vi "bad apple.vi"() -> ()   [LabVIEW 2016]
uses:
  <vilib>/vision/NI_Vision_Development_Module.lvlib
panel:
  out "强度图":sgl[][](graph)
  out "Image 2":T1(plugin-control)
  out "波形图":sgl[][](graph)
  out "Image":T1(plugin-control)
  in  "Stop":bool
  in  "路径":path
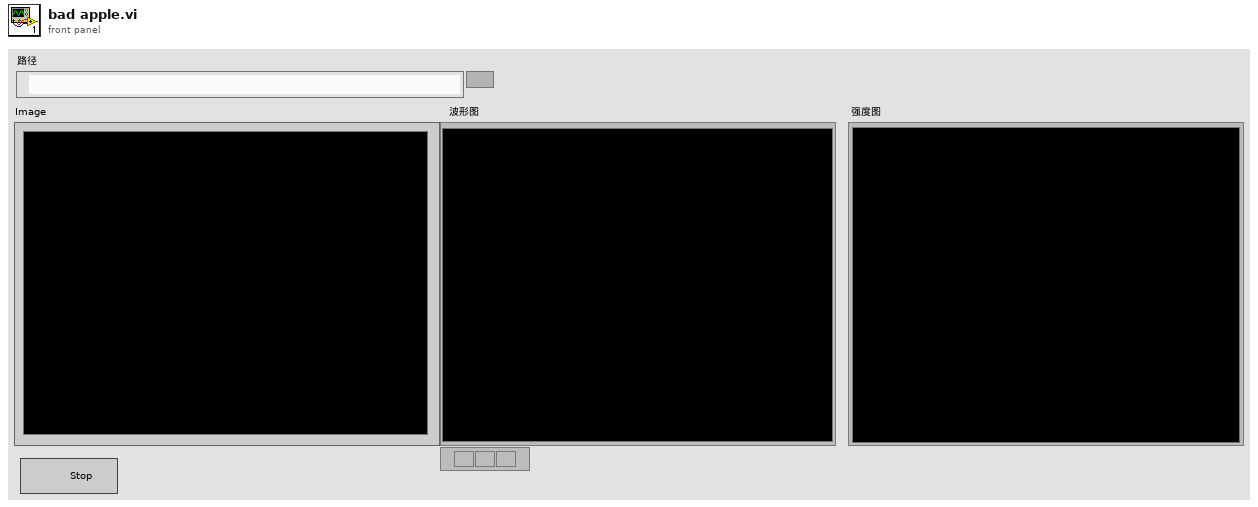
[diagram p1: front panel]
types:
  T1 = typedef "IMAQ Image.ctl" = refnum<image>
  T2 = typedef "Image Type" = u32
  T3 = typedef "IMAQ AVI2 Refnum.ctl" = refnum<k20>
  T4 = cluster{"Width":u32, "Height":u32, "Frames Per Second":u32, "Codec":string, "Has Data":bool}
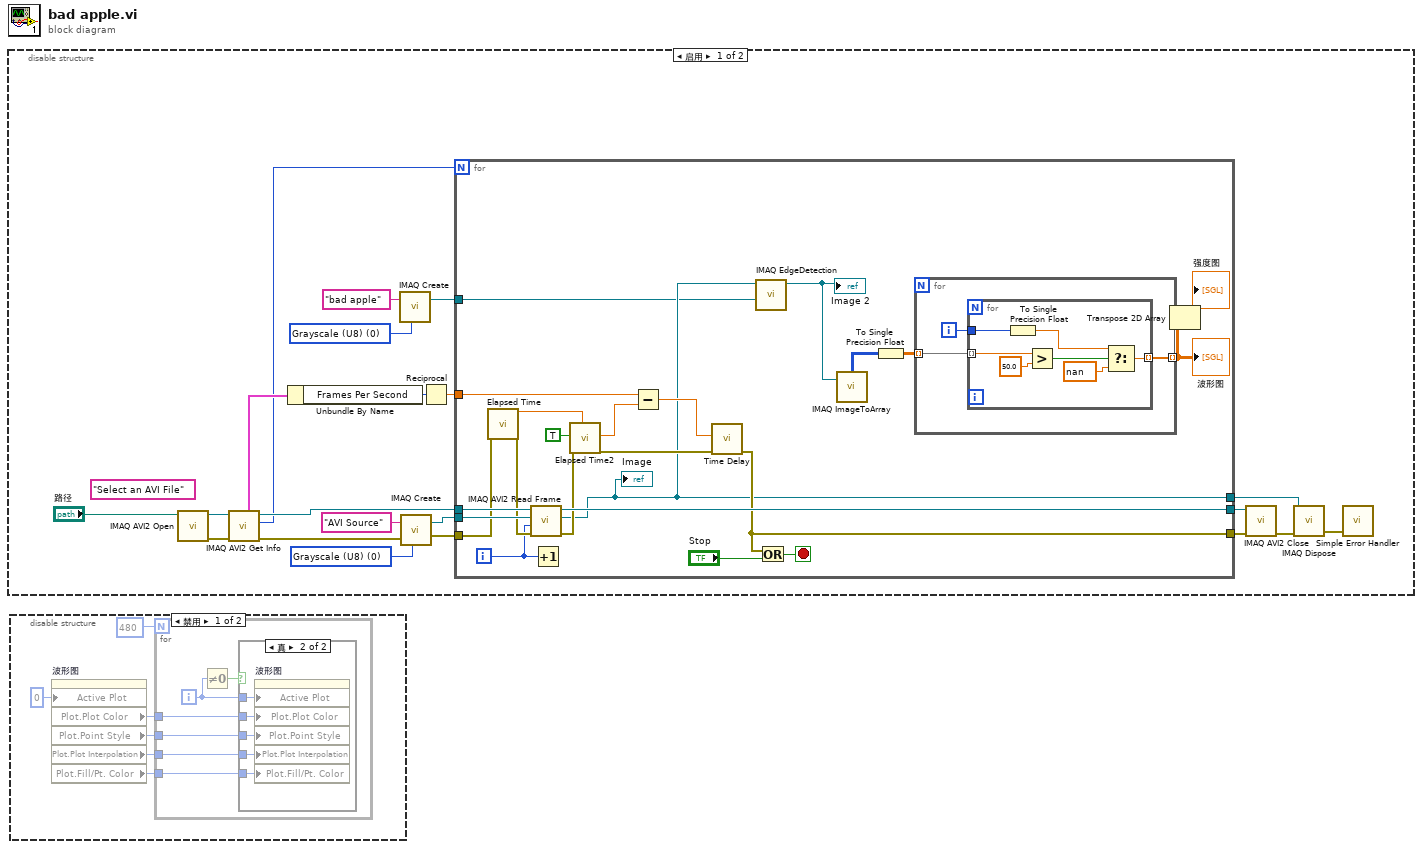
[diagram p0: block diagram]
diagram:
  n1 = disable-structure shown="启用" {
    frame Enabled {
      w3 = T2 0 items=["Grayscale (U8)", "Grayscale (I16)", "Grayscale (SGL)", "Complex (CSG)", "RGB (U32)", "HSL (U32)", "RGB (U64)", "Grayscale (U16)"] ("Image Type")
      w4 = T2 0 items=["Grayscale (U8)", "Grayscale (I16)", "Grayscale (SGL)", "Complex (CSG)", "RGB (U32)", "HSL (U32)", "RGB (U64)", "Grayscale (U16)"] ("Image Type")
      (unwired) "Select an AVI File" ("prompt")
      n2 = call "IMAQ AVI2 Open"("AVI File Path"="路径") -> ("error out"=w18:errorcluster, "AVI Refnum"=w17:T3)  [unwired: 2 in, 7 out]
      n3 = call "IMAQ AVI2 Get Info"("error in (no error)"=w18, "AVI Refnum"=w17) -> ("error out"=w14:errorcluster, "Number of Frames"=w6:u32, "AVI Refnum (duplicate)"=w11:T3, "Frame Data"=w19:T4)  [unwired: 6 out]
      n4 = Unbundle By Name(w19) -> ("Frames Per Second"=w8:u32)
      n5 = call "IMAQ Create"("Image Name"="bad apple", "Image Type"=w3) -> ("New Image"=w1:T1)  [unwired: 3 in, 1 out]
      n6 = call "IMAQ Create"("Image Name"="AVI Source", "Image Type"=w4, "error in (no error)"=w14) -> ("New Image"=w12:T1, "error out"=w13:errorcluster)  [unwired: 1 in, 1 out]
      n7 = Reciprocal(x=w8) -> (1/x=w7:dbl)
      n8 = for {
        N: w6 -> [_]
        tunnel: w12 -> [w43]
        tunnel: [w42] -> w15
        tunnel: [w32] -> w16
        tunnel: w13 -> [w41]
        tunnel: w11 -> [w44]
        tunnel: [w24] -> w9
        tunnel: w7 -> [w39]
        tunnel: w1 -> [w23]
        i -> [w29]
        stop <- w30 stop-if-true
        n9 = call "Elapsed Time"("error in (no error)"=w41) -> ("Present (s)"=w37:dbl, "error out"=w40:errorcluster)  [unwired: 11 in, 6 out]
        n10 = call "IMAQ AVI2 Read Frame"("error in (no error)"=w40, "Frame Number"=w29, "Image"=w43, "AVI Refnum"=w44) -> ("error out"=w35:errorcluster, "Image Out"=w24:T1, "AVI Refnum (duplicate)"=w42:T3)  [unwired: 5 out]
        "Image" <- w24
        n11 = Increment(x=w29) -> ()  [unwired: 1 out]
        n12 = call "Elapsed Time2"("Reset"=TRUE, "error in (no error)"=w35, "Set Start Time (s)"=w37) -> ("Elapsed Time (s)"=w34:dbl, "error out"=w33:errorcluster)  [unwired: 9 in, 6 out]
        n13 = Subtract(x=w39, y=w34) -> (x-y=w38:dbl)
        n14 = call "Time Delay"("error in (no error)"=w33, "Delay Time (s)"=w38) -> ("error out"=w32:errorcluster)  [unwired: 9 in]
        n15 = call "IMAQ EdgeDetection"("Image Dst"=w23, "Image Src"=w24) -> ("Image Dst Out"=w22:T1)  [unwired: 4 in, 5 out]
        "Image 2" <- w22
        n16 = Or(x=w32, y="Stop") -> (x .or. y?=w30:bool)
        n17 = call "IMAQ ImageToArray"("Image"=w22) -> ("Image Pixels (U8)"=w28:u8[][])  [unwired: 3 in, 4 out]
        n18 = To Single Precision Float(number=w28) -> (single precision float=w27:sgl[][])
        n19 = for {
          tunnel: w27 -> [w47] mode=indexing
          tunnel: [w45] -> w26 mode=indexing
          i -> [w46]
          n20 = for {
            tunnel: w47 -> [w52] mode=indexing
            tunnel: w46 -> [w48]
            tunnel: [w49] -> w45 mode=indexing
            n21 = To Single Precision Float(number=w48) -> (single precision float=w51:sgl)
            n22 = Greater?(x=w52, y=sgl 50.0) -> (0:w54:bool)
            n23 = Select(t=w51, s=w54, f=sgl nan) -> (s? t:f=w49:sgl)
          }
        }
        "波形图" <- w26
        n24 = Transpose 2D Array(2D array=w26) -> (transposed array=→"强度图":sgl[][])
      }
      n25 = call "IMAQ AVI2 Close"("error in (no error)"=w16, "AVI Refnum"=w15) -> ("error out"=w10:errorcluster)  [unwired: 9 out]
      n26 = call "IMAQ Dispose"("Image"=w9, "error in (no error)"=w10) -> ("error out"=w20:errorcluster)  [unwired: 1 in, 3 out]
      n27 = call <vilib>:"Simple Error Handler.vi"("error in (no error)"=w20) -> ()  [unwired: 1 in, 8 out]
    }
    frame Disabled {
    }
  }
  n28 = disable-structure shown="禁用" {
    frame Disabled {
      n29 = property on="波形图" class="WFGraph (严格)"("Active Plot"=u32 0 ("活动曲线")) -> ("Plot.Plot Color"=w59:u32, "Plot.Point Style"=w58:u8, "Plot.Plot Interpolation"=w56:u8, "Plot.Fill/Pt. Color"=w55:u32)  [unwired: 2 in, 2 out]
      n30 = for {
        N: 480 -> [_]
        tunnel: w59 -> [w64]
        tunnel: w58 -> [w63]
        tunnel: w56 -> [w62]
        tunnel: w55 -> [w61]
        i -> [w65]
        n31 = Not Equal To 0?(x=w65) -> (x != 0?=w66:bool)
        n32 = case shown="真" w66 {
          tunnel: w65 -> [_ w71]
          tunnel: w64 -> [_ w70]
          tunnel: w63 -> [_ w69]
          tunnel: w62 -> [_ w68]
          tunnel: w61 -> [_ w67]
          frame False {
          }
          frame True {
            n33 = property on="波形图" class="WFGraph (严格)"("Active Plot"=w71, "Plot.Plot Color"=w70, "Plot.Point Style"=w69, "Plot.Plot Interpolation"=w68, "Plot.Fill/Pt. Color"=w67) -> ()  [unwired: 2 in, 2 out]
          }
        }
      }
    }
    frame Enabled {
    }
  }
